vi "View DRV data.vi"(8 "error in (no error)":errorcluster) -> (0 "error out":errorcluster)   [LabVIEW 2018, in "Application.lvlib"]
uses:
  Application.lvlib
  SubVIs/FGV DRV data.ctl
panel:
  out "SC 9":bool caption="ngľn mąch"
  out "SC 8":bool caption="ngľn mąch"
  out "SC 7":bool caption="ngľn mąch"
  out "SC 6":bool caption="ngľn mąch"
  out "SC 5":bool caption="ngľn mąch"
  out "SC 4":bool caption="ngľn mąch"
  out "SC 3":bool caption="ngľn mąch"
  out "SC 2":bool caption="ngľn mąch"
  out "effect min":dbl caption="HIÖU SUĘT"
  out "AC kW (W) min":dbl caption="C¤NG SUĘT AC (Watt)"
  out "DCI(mA) min":dbl caption="§IÖN ¸P DC (mA)"
  out "DCV(Volts) min":dbl caption="§IÖN ¸P DC (Volts)"
  out "pf min":dbl caption="HÖ Sč C¤NG SUĘT"
  out "ACI(mA) min":dbl caption="DßNG §IÖN AC (mA)"
  out "ACV(Volts) min":dbl caption="§iÖn ¸p AC (Volts)"
  out "effect max":dbl caption="HIÖU SUĘT"
  out "AC kW (W) max":dbl caption="C¤NG SUĘT AC (Watt)"
  out "DCI(mA) max":dbl caption="§IÖN ¸P DC (mA)"
  out "DCV(Volts) max":dbl caption="§IÖN ¸P DC (Volts)"
  out "pf  max":dbl caption="HÖ Sč C¤NG SUĘT"
  out "ACI(mA) max":dbl caption="DßNG §IÖN AC (mA)"
  out "ACV(Volts) max":dbl caption="§iÖn ¸p AC (Volts)"
  out "Name":string(combo) caption="TĘN DRIVER"
  out "SAP ID":string
  out "effect":dbl caption="HIÖU SUĘT"
  out "DC kW (W)":dbl caption="C¤NG SUĘT DC (Watt)"
  out "AC kW (W)":dbl caption="C¤NG SUĘT AC (Watt)"
  in  "rst data":bool
  in  "DRV idx(1-60)":i32=1 min=1 max=60
  out "DCI(mA)":dbl caption="§IÖN ¸P DC (mA)"
  out "DCV(Volts)":dbl caption="§IÖN ¸P DC (Volts)"
  out "SC":bool caption="ngľn mąch"
  out "pf":dbl caption="HÖ Sč C¤NG SUĘT"
  out "ACI(mA)":dbl caption="DßNG §IÖN AC (mA)"
  out "ACV(Volts)":dbl caption="§iÖn ¸p AC (Volts)"
  in  "stop":bool
  # "MAX"
  # "MIN"
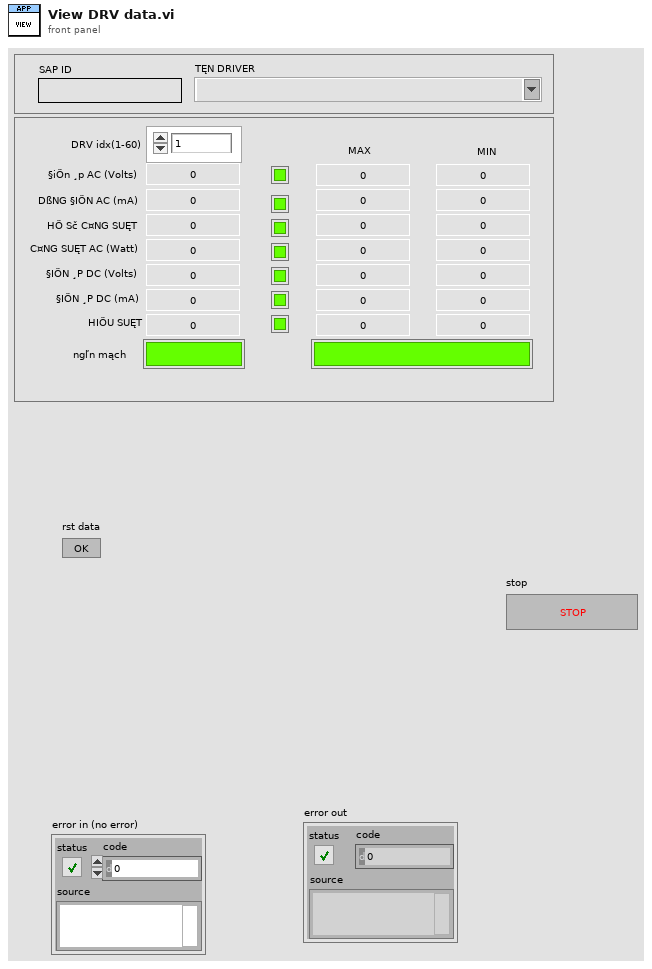
[diagram p1: front panel]
types:
  T1 = typedef "Application.lvlib/FGV DRV data.ctl" = enum16{"Init", "Write", "Read", "Process"}
  T2 = typedef "Application.lvlib/DRV stand.ctl" = cluster{"SAP ID":string, "Name":string, "AC characteristics":cluster{"Voltage":cluster{"Min":dbl, "Max":dbl}, "Current":cluster{"Min":dbl, "Max":dbl}, "kW":cluster{"Min":dbl, "Max":dbl}, "PF":cluster{"Min":dbl, "Max":dbl}}, "DC characteristics":cluster{"Voltage":cluster{"Min":dbl, "Max":dbl}, "Current":cluster{"Min":dbl, "Max":dbl}, "Effect":cluster{"Min":dbl, "Max":dbl}}}
  T3 = cluster{"Voltage":cluster{"Min":dbl, "Max":dbl}, "Current":cluster{"Min":dbl, "Max":dbl}, "kW":cluster{"Min":dbl, "Max":dbl}, "PF":cluster{"Min":dbl, "Max":dbl}}
  T4 = cluster{"Voltage":cluster{"Min":dbl, "Max":dbl}, "Current":cluster{"Min":dbl, "Max":dbl}, "Effect":cluster{"Min":dbl, "Max":dbl}}
  T5 = typedef "Application.lvlib/DRV cluster 2.ctl" = cluster{"Shorted Circuit":bool, "AC voltage(volts)":dbl, "AC Current (mA)":dbl, "AC kW (W)":dbl, "AC pF ":dbl, "DC Voltage (Volts)":dbl, "DC Current (mA)":dbl, "DC kW (W)":dbl, "DRV Fail/Pass (T)":bool}
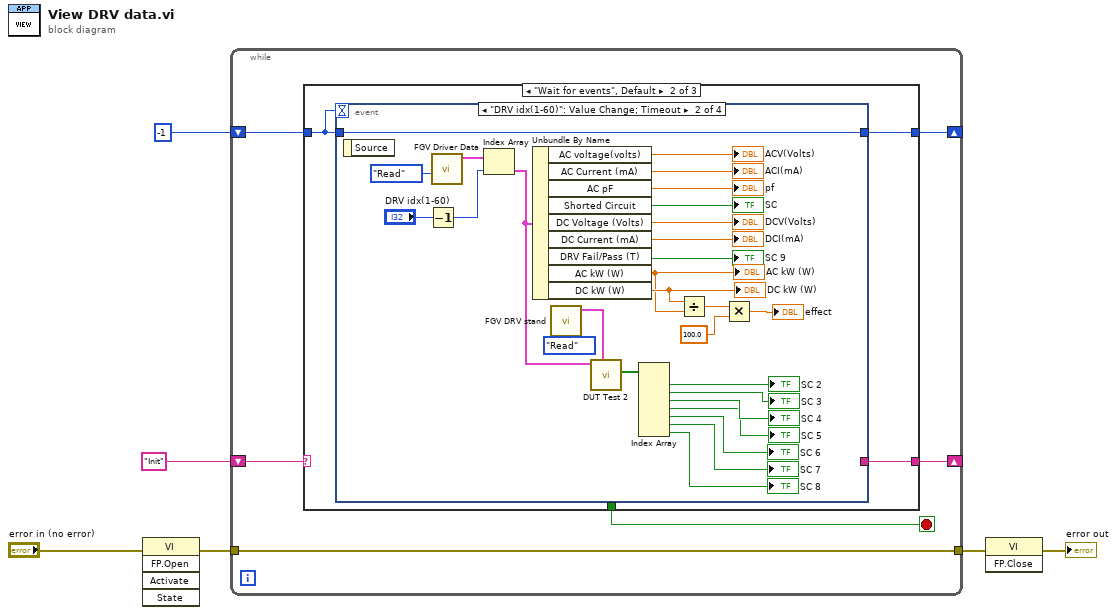
[diagram p0: block diagram]
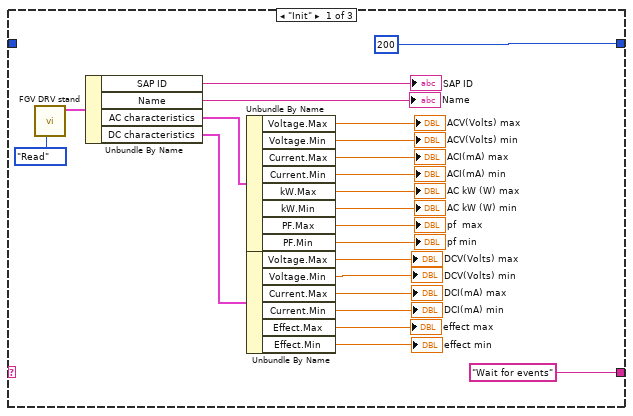
[diagram p2: hidden frame]
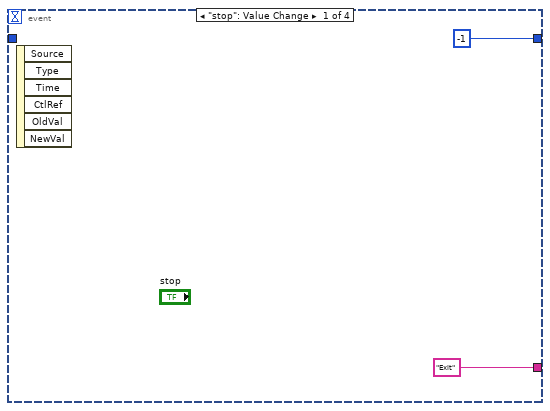
[diagram p3: hidden frame]
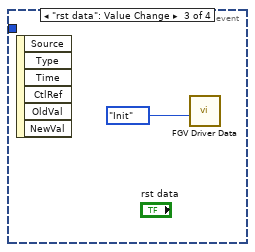
[diagram p4: hidden frame]
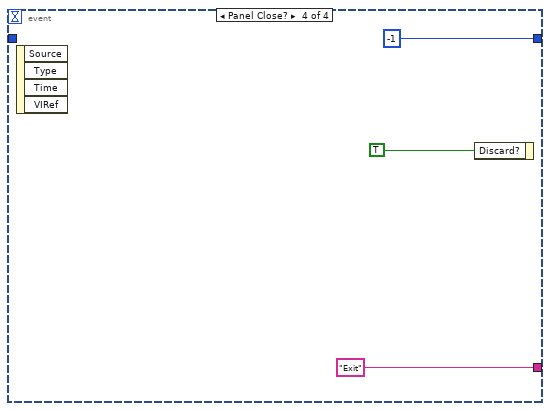
[diagram p5: hidden frame]
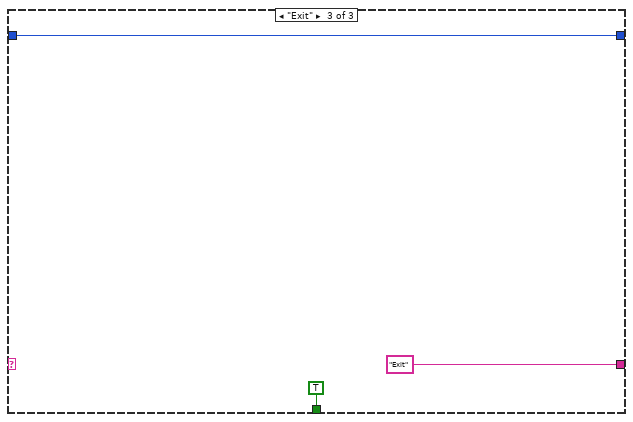
[diagram p6: hidden frame]
diagram:
  n1 = invoke class="VI" method="FP.Open"(error in="error in (no error)") -> (error out=w6:errorcluster)  [unwired: 4 in, 4 out]
  n2 = while {
    tunnel: w6 -> [w11]
    tunnel: [w11] -> w5
    shift-right: [w9] -> _
    shift-left: "Init" -> [w10]
    shift-right: [w7] -> _
    shift-left: -1 -> [w8]
    stop <- w12 stop-if-true
    n3 = case shown="\"Wait for events\", Default" w10 {
      tunnel: [_ _ TRUE] -> w12
      tunnel: ["Wait for events" w35 "Exit"] -> w9
      tunnel: w8 -> [_ w36 w71]
      tunnel: [200 w37 w71] -> w7
      frame "Init" {
        n4 = call "FGV DRV stand.vi"("Enum"=enum16{"Write", "Read"}."Read") -> ("DRV stand out"=w33:T2)  [unwired: 10 in]
        n5 = Unbundle By Name(w33) -> ("SAP ID"=→"SAP ID":string, "Name"=→"Name":string, "AC characteristics"=w29:T3, "DC characteristics"=w20:T4)
        n6 = Unbundle By Name(w29) -> ("Voltage.Max"=→"ACV(Volts) max":dbl, "Voltage.Min"=→"ACV(Volts) min":dbl, "Current.Max"=→"ACI(mA) max":dbl, "Current.Min"=→"ACI(mA) min":dbl, "kW.Max"=→"AC kW (W) max":dbl, "kW.Min"=→"AC kW (W) min":dbl, "PF.Max"=→"pf  max":dbl, "PF.Min"=→"pf min":dbl)
        n7 = Unbundle By Name(w20) -> ("Voltage.Max"=→"DCV(Volts) max":dbl, "Voltage.Min"=→"DCV(Volts) min":dbl, "Current.Max"=→"DCI(mA) max":dbl, "Current.Min"=→"DCI(mA) min":dbl, "Effect.Max"=→"effect max":dbl, "Effect.Min"=→"effect min":dbl)
      }
      frame "Wait for events", Default {
        n8 = event shown="[1] \"DRV idx(1-60)\": Value Change;  Timeout" {
          selector: _ -> [_ _ _ _]
          dyn-events: _ -> [_ _ _ _]
          timeout: w36 -> [_ _ _ _]
          tunnel: [-1 w52 _ -1] -> w37
          tunnel: w36 -> [_ w52 _ _]
          tunnel: ["Exit" _ _ "Exit"] -> w35
          event "stop": Value Change {
            n9 = event-data() -> ()  [unwired: 1 in, 6 out]
          }
          event "DRV idx(1-60)": Value Change; Timeout {
            (unwired) enum16{"Write", "Read"}."Read" ("Enum")
            n10 = event-data() -> ()  [unwired: 1 in, 1 out]
            n11 = Decrement(x="DRV idx(1-60)") -> (x-1=w58:i32)
            n12 = call "FGV Driver Data.vi"("FGV enum"=FGV_DRV_data."Read" ("FGV DRV data enum")) -> ("60 DRV data"=w50:T5[])  [unwired: 7 in, 3 out]
            n13 = Index Array(array=w50, index=w58) -> (element=w49:T5)
            n14 = Unbundle By Name(w49) -> ("AC voltage(volts)"=→"ACV(Volts)":dbl, "AC Current (mA)"=→"ACI(mA)":dbl, "AC pF"=→"pf":dbl, "Shorted Circuit"=→"SC":bool, "DC Voltage (Volts)"=→"DCV(Volts)":dbl, "DC Current (mA)"=→"DCI(mA)":dbl, "DRV Fail/Pass (T)"=→"SC 9":bool, "AC kW (W)"=w56:dbl, "DC kW (W)"=w57:dbl)
            "AC kW (W)" <- w56
            "DC kW (W)" <- w57
            n15 = call "FGV DRV stand.vi"() -> ("DRV stand out"=w51:T2)  [unwired: 11 in]
            n16 = call "DUT Test 2.vi"("DRV stand"=w51, "DRV data"=w49) -> ("details"=w47:bool[])  [unwired: 7 in, 2 out]
            n17 = Index Array(array=w47) -> (element #1=→"SC 2":bool, element #2=→"SC 3":bool, element #3=→"SC 4":bool, element #4=→"SC 5":bool, element #5=→"SC 6":bool, element #6=→"SC 7":bool, element #7=→"SC 8":bool)  [unwired: 7 in]
            n18 = Divide(x=w57, y=w56) -> (x/y=w54:dbl)
            n19 = Multiply(x=w54, y=100.0) -> (x*y=→"effect":dbl)
          }
          event "rst data": Value Change {
            n20 = event-data() -> ()  [unwired: 1 in, 6 out]
            n21 = call "FGV Driver Data.vi"("FGV enum"=FGV_DRV_data."Init" ("FGV DRV data enum")) -> ()  [unwired: 7 in, 4 out]
          }
          event Panel Close? {
            n22 = event-data() -> ()  [unwired: 1 in, 4 out]
            n23 = event-data("Discard?"=TRUE) -> ()  [unwired: 1 in, 1 out]
          }
        }
      }
      frame "Exit" {
      }
    }
  }
  n24 = invoke class="VI" method="FP.Close"(error in=w5) -> (error out=→"error out":errorcluster)  [unwired: 2 in, 2 out]
